vi "Validate Database.vi"(8 "error in (no error)":errorcluster, 11 "Paquetes Disponibles in":refnum<class "Paquetes Disponibles.lvclass">) -> (0 "error out":errorcluster, 3 "Paquetes Disponibles out":refnum<class "Paquetes Disponibles.lvclass">)   [LabVIEW 2020, in "Paquetes Disponibles.lvlib" / "Paquetes Disponibles.lvclass"]
uses:
  Paquetes Disponibles.lvclass
  C:/Program Files (x86)/National Instruments/LabVIEW 2020/vi.lib/ActorFramework/Actor/Actor.lvclass
  <vilib>/ActorFramework/Actor/Actor.lvclass/Actor.ctl
  <vilib>/ActorFramework/Message Enqueuer/Message Enqueuer.lvclass/Message Enqueuer.ctl
  Paquetes Disponibles Messages/Timestamp Msg/Timestamp Msg.lvclass/Timestamp Msg.ctl
  <vilib>/ActorFramework/Message Enqueuer/Init from Existing Queue.vi
  <vilib>/ActorFramework/Message Enqueuer/Enqueue.vi
  Paquetes Disponibles Messages/Timestamp Msg/Timestamp Msg.lvclass
  C:/Program Files (x86)/National Instruments/LabVIEW 2020/vi.lib/ActorFramework/Message/Message.lvclass
  <vilib>/ActorFramework/Message Priority Queue/Priority Enqueue.vi
  <vilib>/ActorFramework/Message Enqueuer/Message Enqueuer.lvclass
  <vilib>/ActorFramework/Actor/Actor.lvclass
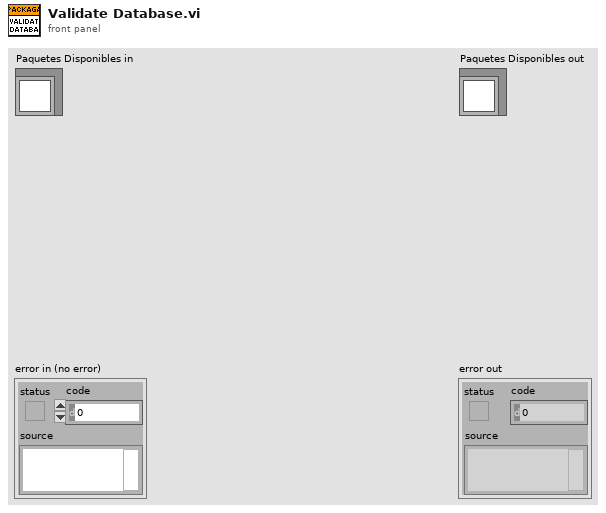
[diagram p1: front panel]
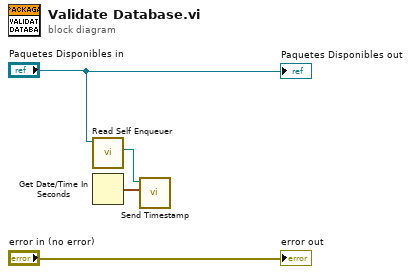
[diagram p0: block diagram]
diagram:
  n1 = call <vilib>:"Read Self Enqueuer.vi"("Actor"="Paquetes Disponibles in") -> ("Self Enqueuer"=w2:refnum<class "Message Enqueuer.lvclass">)  [unwired: 10 in]
  n2 = Get Date/Time In Seconds() -> (seconds since 1Jan1904=w3:timestamp)
  n3 = call "Send Timestamp.vi"("First Time"=w3, "Message Enqueuer"=w2) -> ()  [unwired: 8 in, 2 out]
  "error out" <- "error in (no error)"
  "Paquetes Disponibles out" <- "Paquetes Disponibles in"
